vi "stop.vi"(8 "error in":errorcluster, 10 "NATS Client":refnum<class "NATS Client.lvclass">, 11 "NATS Subscription":refnum<class "NATS Subscription.lvclass">) -> (0 "error out":errorcluster)   [LabVIEW 2024, in "NAT Subscription.lvlib" / "NATS Subscription.lvclass"]
uses:
  NATS Subscription.lvclass
  NATS Client/NATS Client.lvclass
  NATS Subscription.lvclass/NATS Subscription.ctl
  get reply queue.vi
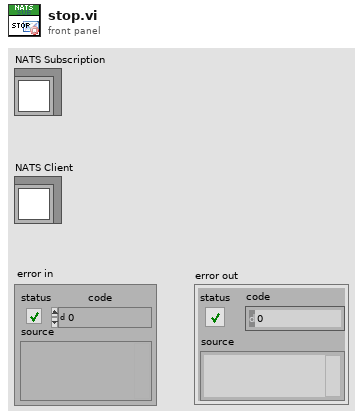
[diagram p1: front panel]
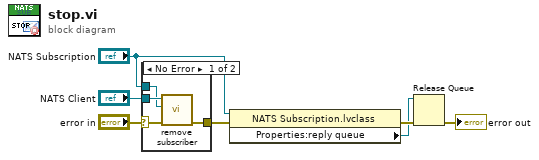
[diagram p0: block diagram]
diagram:
  n1 = case shown="No Error" "error in" {
    selector: "error in" -> [w10 w12]
    tunnel: [w11 w12] -> w6
    tunnel: "NATS Client" -> [w9 _]
    tunnel: "NATS Subscription" -> [w8 _]
    frame No Error {
      n2 = call "remove subscriber.vi"("error in"=w10, "NATS Subscription"=w8, "NATS Client in"=w9) -> ("error out"=w11:errorcluster)  [unwired: 7 in, 1 out]
    }
    frame Error {
    }
  }
  n3 = property class="NATS Subscription.lvclass"(reference="NATS Subscription", error in=w6) -> (error out=w4:errorcluster, "Properties:reply queue"=w1:refnum<queue>)  [unwired: 1 out]
  n4 = Release Queue(queue=w1, error in (no error)=w4) -> (error out=→"error out":errorcluster)  [unwired: 1 in, 2 out]
